vi "Arm Setpoint.vi"(0 "Arm Control":dbl(slide) scale=0.0..10.0, 1 "Setpoint Angle":dbl, 2 "Loop Disable":bool) -> ()   [LabVIEW 2023]
uses:
  <vilib>/Rock Robotics/Network Tables/NT Write Float.vi
  <vilib>/addons/control/pid/pid.llb/PID (DBL).vi
  <vilib>/addons/control/pid/NI_PID_pid.lvlib
panel:
  in  "PID gains":T1={"proportional gain (Kc)"=0.017, "integral time (Ti, min)"=0.08, "derivative time (Td, min)"=1e-05} {"derivative time (Td, min)" format="%.6f"; "integral time (Ti, min)" format="%.6f"; "proportional gain (Kc)" format="%.6f"}
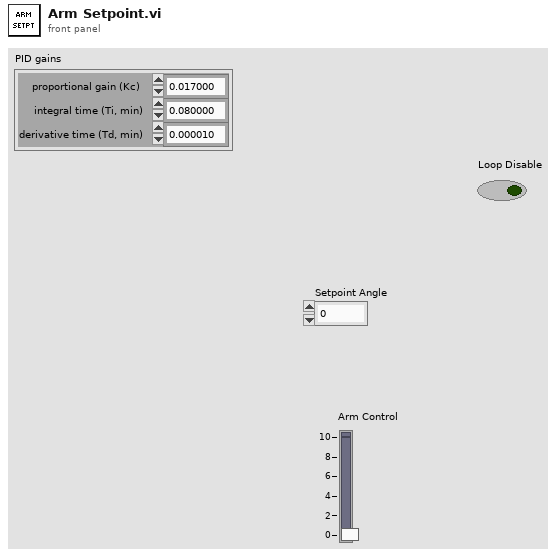
[diagram p1: front panel]
types:
  T1 = cluster{"proportional gain (Kc)":dbl, "integral time (Ti, min)":dbl, "derivative time (Td, min)":dbl}
  T2 = cluster{"Yaw":dbl, "Roll":dbl, "Pitch":dbl, "Heading":dbl, "Fused Heading":dbl}
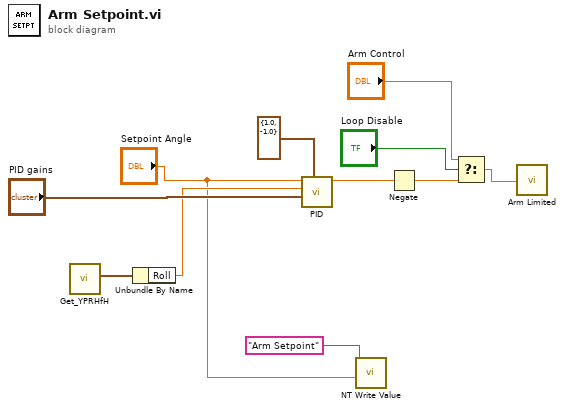
[diagram p0: block diagram]
diagram:
  n1 = call <vilib>:"Get_YPRHfH.vi"() -> ("YRPHfH"=w10:T2)  [unwired: 11 in]
  n2 = Unbundle By Name(w10) -> ("Roll"=w9:dbl)
  n3 = call-poly <vilib>:"PID.vi"("output range"=cluster{"output high":dbl, "output low":dbl} {"output high"=1.0, "output low"=-1.0}, "PID gains"="PID gains", "process variable"=w9, "setpoint"="Setpoint Angle") -> ("output"=w7:dbl)  [unwired: 6 in, 1 out]
  n4 = call-poly <vilib>:"NT Write Value.vi"("value"="Setpoint Angle", "name"="Arm Setpoint") -> ()  [unwired: 9 in, 1 out]
  n5 = Negate(x=w7) -> (-x=w4:dbl)
  n6 = Select(t="Arm Control", s="Loop Disable", f=w4) -> (s? t:f=w3:dbl)
  n7 = call "Arm Limited.vi"("Arm Command"=w3) -> ()  [unwired: 1 out]
